vi "Write DUT Setup Parameters.vi"(8 "error in (no error)":errorcluster, 10 "DUT Setup Parameters":T1[](array[typedef]), 11 "QPA Measurement in":refnum<class "QPA Measurement.lvclass">=refnum) -> (0 "error out":errorcluster, 3 "QPA Measurement out":refnum<class "QPA Measurement.lvclass">)   [LabVIEW 2016, in "QPA Measurement.lvlib" / "QPA Measurement.lvclass"]
uses:
  QPA Measurement.lvclass
  Controls/Parameter.ctl
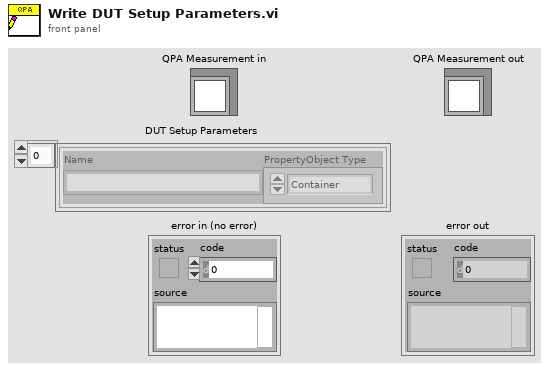
[diagram p1: front panel]
types:
  T1 = typedef "QPA Measurement.lvlib/QPA Measurement.lvclass/Parameter.ctl" = cluster{"Name":string, "PropertyObject Type":enum16{"Container", "String", "Boolean", "Number", "NamedType", "Reference", "Array"}}
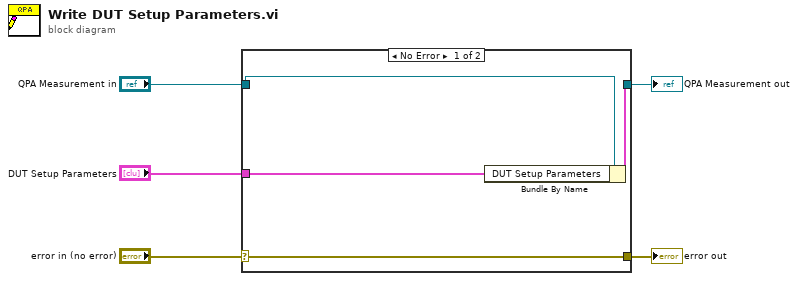
[diagram p0: block diagram]
diagram:
  n1 = case shown="No Error" "error in (no error)" {
    selector: "error in (no error)" -> [w9 w10]
    tunnel: [w9 w10] -> w4
    tunnel: [w7 w11] -> w2
    tunnel: "QPA Measurement in" -> [w8 w11]
    tunnel: "DUT Setup Parameters" -> [w6 _]
    frame No Error {
      n2 = Bundle By Name(cluster=w8, "DUT Setup Parameters"=w6) -> (w7:cluster{})
    }
    frame Error {
    }
  }
  "error out" <- w4
  "QPA Measurement out" <- w2
